vi "Orbitron_ConvertTime2Excelvi.vi"(3 "OrbitronTimeDateString":string="20210106190936") -> (0 "JD&ModJD":string, 1 "DateTime":string)   [LabVIEW 2013]
panel:
  out "ModJD 2":string
  out "ModifiedJulian":dbl format="%#_17g"
  out "PartOfDay":dbl
  out "JDay":dbl
  out "JD":dbl format="%#.15g"
  out "Time":string
  out "Date":string
  out "sec":string
  out "min":string
  out "hr":string
  out "Month":string
  out "Day":string
  out "yr":string
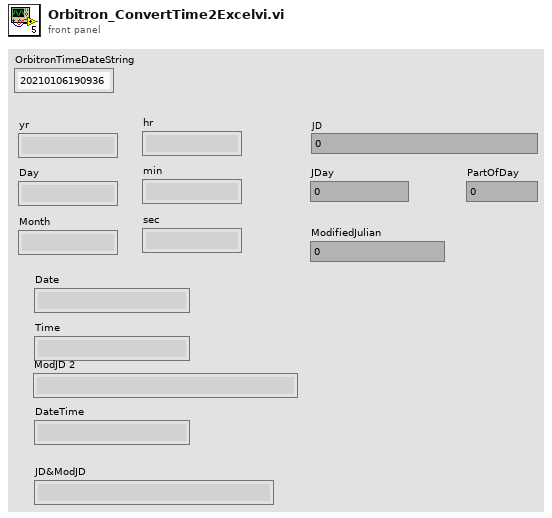
[diagram p1: front panel]
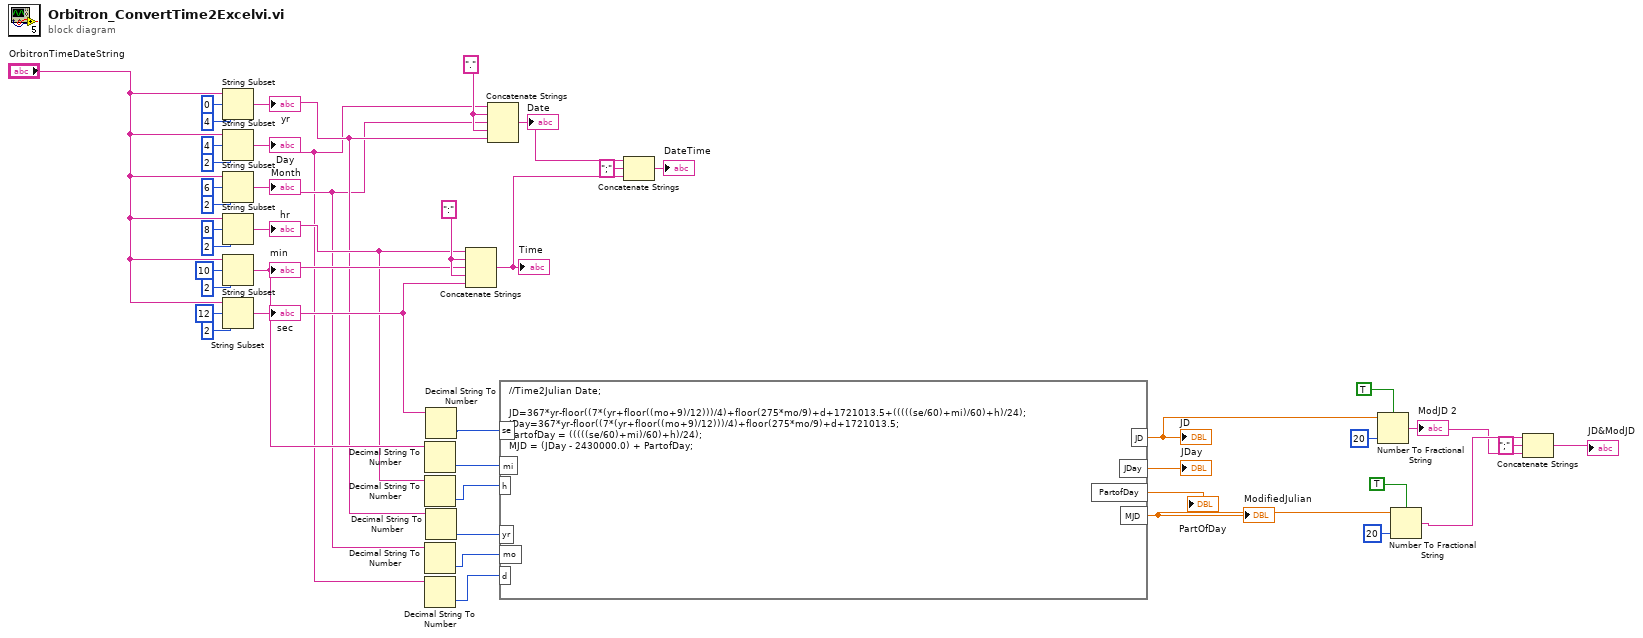
[diagram p0: block diagram]
diagram:
  w29 = ":" ("string")
  w30 = "." ("string")
  n1 = String Subset(string="OrbitronTimeDateString", offset (0)=0, length (rest)=4 ("length (rest)")) -> (substring=w15:string)
  "yr" <- w15
  n2 = String Subset(string="OrbitronTimeDateString", offset (0)=4, length (rest)=2 ("length (rest)")) -> (substring=w11:string)
  "Day" <- w11
  n3 = String Subset(string="OrbitronTimeDateString", offset (0)=6, length (rest)=2 ("length (rest)")) -> (substring=w13:string)
  "Month" <- w13
  n4 = String Subset(string="OrbitronTimeDateString", offset (0)=8, length (rest)=2 ("length (rest)")) -> (substring=w17:string)
  "hr" <- w17
  n5 = String Subset(string="OrbitronTimeDateString", offset (0)=10, length (rest)=2 ("length (rest)")) -> (substring=w20:string)
  "min" <- w20
  n6 = String Subset(string="OrbitronTimeDateString", offset (0)=12, length (rest)=2 ("length (rest)")) -> (substring=w21:string)
  "sec" <- w21
  n7 = Decimal String To Number(string=w20) -> (number=w19:i32)  [unwired: 2 in, 1 out]
  n8 = Decimal String To Number(string=w17) -> (number=w18:i32)  [unwired: 2 in, 1 out]
  n9 = Decimal String To Number(string=w13) -> (number=w14:i32)  [unwired: 2 in, 1 out]
  n10 = Decimal String To Number(string=w11) -> (number=w12:i32)  [unwired: 2 in, 1 out]
  n11 = Decimal String To Number(string=w21) -> (number=w22:i32)  [unwired: 2 in, 1 out]
  n12 = Decimal String To Number(string=w15) -> (number=w16:i32)  [unwired: 2 in, 1 out]
  n13 = Concatenate Strings(w17, w29, w20, w29, w21) -> (w27:string)
  "Time" <- w27
  n14 = Concatenate Strings(w11, w30, w13, w30, w15) -> (w28:string)
  "Date" <- w28
  n15 = formula code="//Time2Julian Date;\n\nJD=367*yr-floor((7*(yr+floor((mo+9)/12)))/4)+floor(275*mo/9)+d+1721013.5+(((((se/60)+mi)/60)+h)/24);\nJDay=367*yr-floor((7*(yr+floor((mo+9)/12)))/4)+floor(275*mo/9)+d+1721013.5;\nPartofDay = (((((se/60)+mi)/60)+h)/24);\nMJD = (JDay - 2430000.0) + PartofDay;"("yr"=w16, "mo"=w14, "d"=w12, "h"=w18, "mi"=w19, "se"=w22) -> ("JD"=w5:dbl, "JDay"=→"JDay":dbl, "PartofDay"=→"PartOfDay":dbl, "MJD"=w10:dbl)
  "JD" <- w5
  "ModifiedJulian" <- w10
  n16 = Concatenate Strings(w28, ";" ("string"), w27) -> (→"DateTime":string)
  n17 = Number To Fractional String(use system decimal point (T)=TRUE, number=w5, precision (6)=i16 20) -> (F-format string=w2:string)  [unwired: 1 in]
  "ModJD 2" <- w2
  n18 = Number To Fractional String(use system decimal point (T)=TRUE, number=w10, precision (6)=i16 20) -> (F-format string=w4:string)  [unwired: 1 in]
  n19 = Concatenate Strings(w4, ";" ("string"), w2) -> (→"JD&ModJD":string)
